vi "test.vi"() -> ()   [LabVIEW 2012]
uses:
  OLD_apparatus_VI/VI/Clearing_mode.ctl
  OLD_apparatus_VI/VI/Readout_mode.ctl
  OLD_apparatus_VI/VI/ADC_gain.ctl
  OLD_apparatus_VI/VI/Image_type.ctl
panel:
  out "Array":T1(array[cluster])
  in  "Image type":T2=7 items=["8 bit signed"=1, "16 bit signed"=2, "32 bit signed"=3, "32 bit floating"=4, "64 bit floating"=5, "8 bit unsigned"=6, "16 bit unsigned"=7, "32 bit unsigned"=8]
  in  "Number of Images":u32=10
  in  "Acquire / Focus Flag":u32=1
  in  "stop":bool=TRUE
  out "Number of Cameras":i32
  out "img":u16[][](graph)
  out "Ydim":u32
  out "Xdim":u32
  out "Camera Handle":u32
  out "error out":errorcluster
  out "Image Handle":u32
  in  "ADC Gain":T3=-1 items=["Use current ADC"=-1, "Use the fastest ADC"=-2, "Use the slowest ADC"=-3]
  in  "FastADC":bool
  in  "ReadoutMode":T4=2.0 caption="Readout Mode" items=["Normal readout"=1.0, "Frame transfer readout"=2.0, "MPP readout"=3.0, "Frame transfer MPP"=4.0, "Alternate timing for normal readout"=5.0, "Alternate timing for frame transfer"=6.0, "Alternate timing for MPP"=7.0, "Alternate timing for frame transfer MPP"=8.0, "Interline"=9.0]
  in  "ClearMode":T5=1.0 caption="Clearing Mode" items=["Clear never"=1.0, "Clear pre-exposure"=2.0, "Clear pre-sequence"=3.0, "Clear post-sequence"=4.0, "Clear pre- and post-sequence"=5.0, "Clear pre-exposure and post-sequence"=6.0]
  in  "EMGain":dbl=3500.0 caption="EM Gain" format="%.2f"
  in  "Exposure (sec)":dbl=0.01 format="%.3f"
  in  "Temperature":dbl=-70.0 format="%.2f"
  in  "error in (no error)":errorcluster
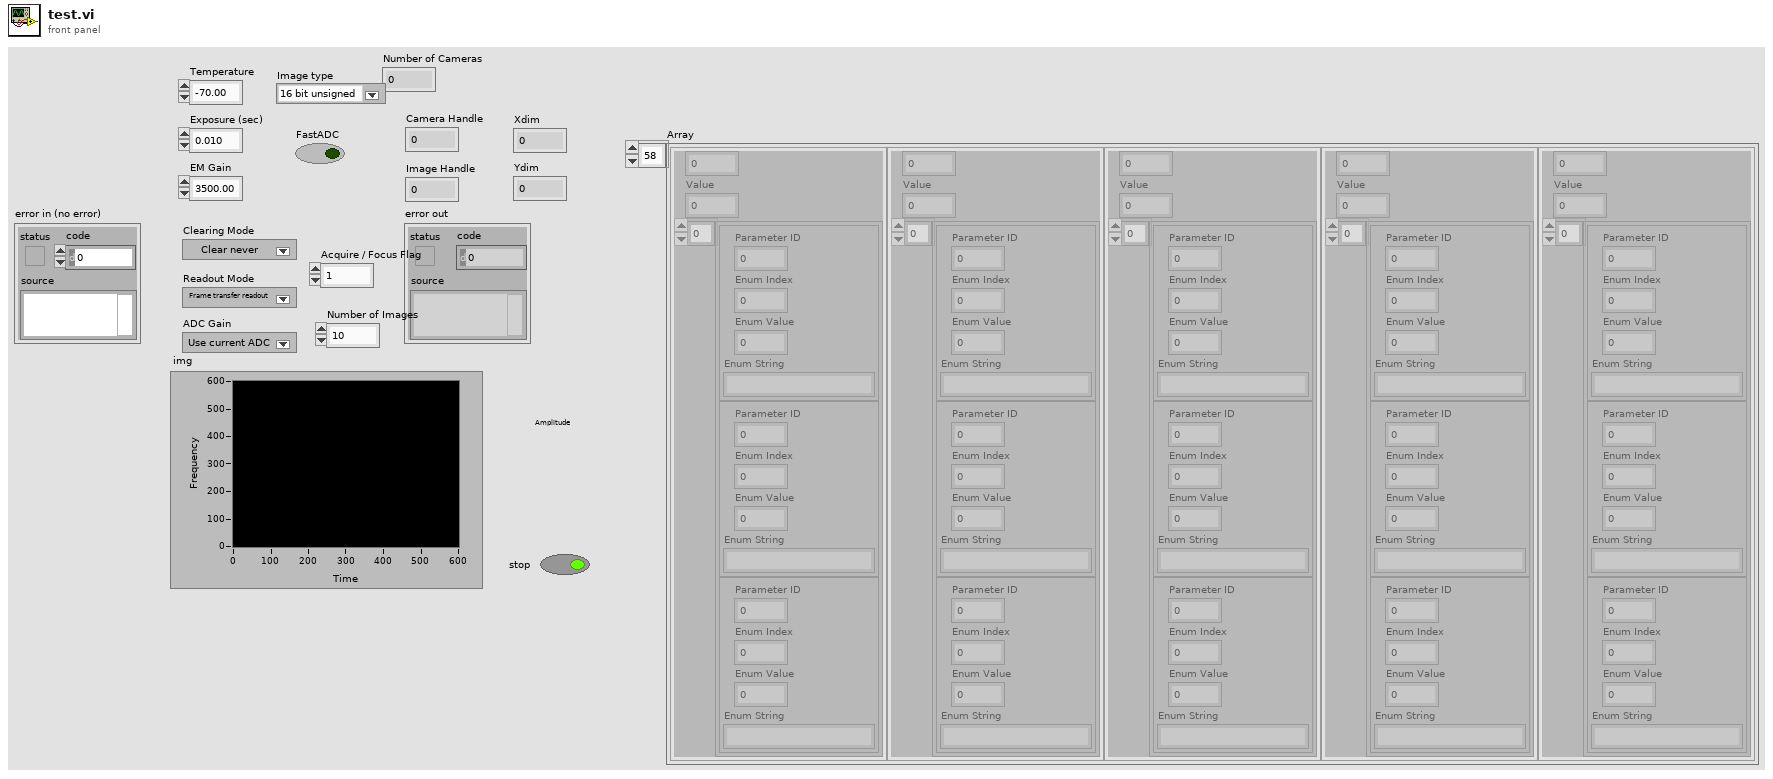
[diagram p1: front panel]
types:
  T1 = cluster{i32, "Value":dbl, cluster{"Parameter ID":u32, "Enum Index":u32, "Enum Value":dbl, "Enum String":string}[]}[]
  T2 = typedef "Image_type.ctl" = u32
  T3 = typedef "ADC_gain.ctl" = i32
  T4 = typedef "Readout_mode.ctl" = dbl
  T5 = typedef "Clearing_mode.ctl" = dbl
  T6 = cluster{"Parameter ID":u32, "Enum Index":u32, "Enum Value":dbl, "Enum String":string}
  T7 = cluster{i32, "Value":dbl, cluster{"Parameter ID":u32, "Enum Index":u32, "Enum Value":dbl, "Enum String":string}[]}
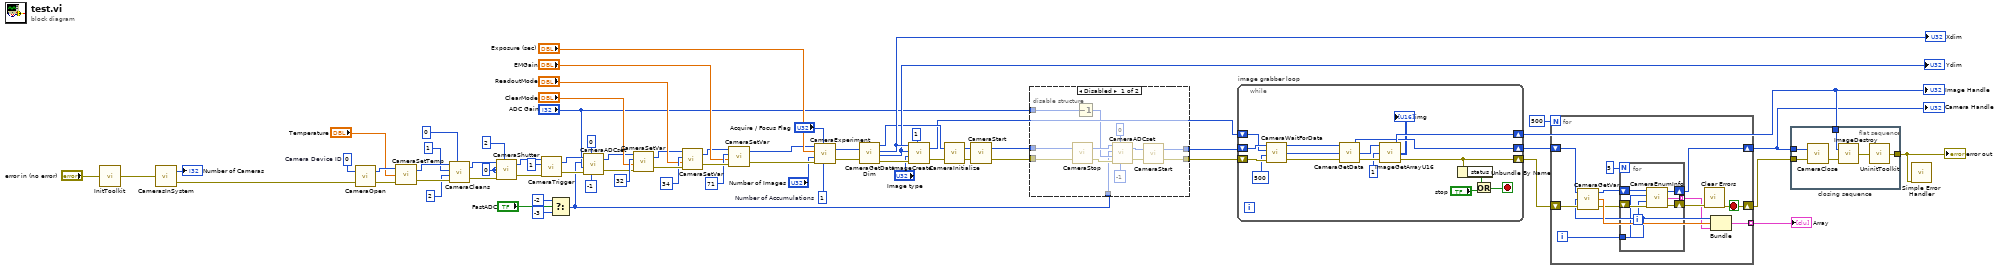
[diagram p0: block diagram]
diagram:
  w14 = u32 1  # Number of Accumulations
  w70 = u32 0  # Camera Device ID
  w60 = u32 0 ("Shutter Comp Time: Pre Open")
  n1 = call <userlib>:"InitToolkit.vi"("error in"="error in (no error)") -> ("error out"=w20:errorcluster)
  n2 = call <userlib>:"CamerasInSystem.vi"("error in"=w20) -> ("Number of Cameras"=→"Number of Cameras":i32, "error out"=w19:errorcluster)
  n3 = call <userlib>:"CameraOpen.vi"("error in"=w19, "Camera Device ID"=w70) -> ("error out"=w68:errorcluster, "Camera Handle"=w69:u32)
  n4 = call <userlib>:"CameraSetTemp.vi"("error in (no error)"=w68, "Temperature"="Temperature", "Camera Handle"=w69) -> ("error out"=w64:errorcluster, "Camera Handle"=w63:u32)
  n5 = call <userlib>:"CameraCleans.vi"("Camera Handle"=w63, "Number of Clears"=u32 1, "Number of Strips Per Clear"=u32 2, "error in"=w64, "Continuous Clears"=u32 0) -> ("Camera Handle"=w65:u32, "error out"=w66:errorcluster)
  n6 = call <userlib>:"CameraShutter.vi"("Camera Handle"=w65, "Shutter Comp Time: Pre Open"=w60, "Shutter Comp Time: Post Open"=w60, "error in"=w66, "Shutter State"=u32 2) -> ("Camera Handle"=w57:u32, "error out"=w58:errorcluster)
  n7 = call <userlib>:"CameraTrigger.vi"("error in"=w58, "Timing Mode"=u32 1, "Camera Handle"=w57) -> ("error out"=w43:errorcluster, "Camera Handle"=w44:u32)  [unwired: 1 in]
  n8 = Select(t=-2 ("Fastest\nADC"), s="FastADC", f=-3 ("Slowest\nADC")) -> (s? t:f=w22:i32)
  n9 = call <userlib>:"CameraADCset.vi"("ADC offset"=-1, "Read Out port"=0, "error in (no error)"=w43, "ADC Gain"="ADC Gain", "ADC Speed"=w22, "Camera Handle"=w44) -> ("error out"=w42:errorcluster, "Camera Handle"=w41:u32)
  n10 = call <userlib>:"CameraSetVar.vi"("error in"=w42, "Value"="ClearMode", "Parameter ID"=u32 32, "Camera Handle"=w41) -> ("error out"=w51:errorcluster, "CameraHandle"=w32:u32)
  n11 = call <userlib>:"CameraSetVar.vi"("error in"=w51, "Value"="ReadoutMode", "Parameter ID"=u32 34, "Camera Handle"=w32) -> ("error out"=w47:errorcluster, "CameraHandle"=w31:u32)
  n12 = call <userlib>:"CameraSetVar.vi"("error in"=w47, "Value"="EMGain", "Parameter ID"=u32 71, "Camera Handle"=w31) -> ("error out"=w38:errorcluster, "CameraHandle"=w37:u32)
  n13 = call <userlib>:"CameraExperiment.vi"("Number of Accumulations"=w14, "Acquire / Focus Flag"="Acquire / Focus Flag", "error in"=w38, "Number of Images"="Number of Images", "Exposure (sec)"="Exposure (sec)", "Camera Handle"=w37) -> ("error out"=w55:errorcluster, "Camera Handle"=w10:u32)
  n14 = call <userlib>:"CameraGetDataDim.vi"("Camera Handle"=w10, "error in"=w55) -> ("Camera Handle"=w9:u32, "Xdim"=w34:u32, "Ydim"=w33:u32, "error out"=w36:errorcluster)
  "Xdim" <- w34
  "Ydim" <- w33
  n15 = call <userlib>:"ImageCreate.vi"("X dimension"=w34, "Y dimension"=w33, "Data Type"="Image type", "error in"=w36, "Number Of Frames"=u32 1) -> ("Image Handle"=w7:u32, "error out"=w12:errorcluster)
  n16 = call <userlib>:"CameraInitialize.vi"("error in"=w12, "Camera Handle"=w9) -> ("error out"=w11:errorcluster, "Camera Handle"=w13:u32)
  n17 = call <userlib>:"CameraStart.vi"("error in"=w11, "Camera Handle"=w13) -> ("error out"=w27:errorcluster, "Camera Handle"=w26:u32)
  n18 = disable-structure shown="Disabled" {
    disable-tunnel: w27 -> [w80 w85]
    disable-tunnel: w26 -> [w79 w86]
    disable-tunnel: [w78 w85] -> w25
    disable-tunnel: [w77 w86] -> w24
    disable-tunnel: "ADC Gain" -> [w74 _]
    disable-tunnel: w22 -> [w72 _]
    frame Disabled {
      n19 = call <userlib>:"CameraStop.vi"("error in"=w80, "Camera Handle"=w79) -> ("error out"=w81:errorcluster, "Camera Handle"=w82:u32)
      n20 = Decrement(x=w74) -> (x-1=w73:T3)
      n21 = call <userlib>:"CameraADCset.vi"("ADC offset"=-1, "Read Out port"=0, "error in (no error)"=w81, "ADC Gain"=w73, "ADC Speed"=w72, "Camera Handle"=w82) -> ("error out"=w76:errorcluster, "Camera Handle"=w75:u32)
      n22 = call <userlib>:"CameraStart.vi"("error in"=w76, "Camera Handle"=w75) -> ("error out"=w78:errorcluster, "Camera Handle"=w77:u32)
    }
    frame Enabled {
    }
  }
  n23 = while "image grabber loop" {
    shift-right: [w102] -> w21
    shift-left: w7 -> [w93]
    shift-right: [w101] -> w6
    shift-left: w24 -> [w97]
    shift-right: [w103] -> w4
    shift-left: w25 -> [w96]
    stop <- w99 stop-if-true
    n24 = call <userlib>:"CameraWaitForData.vi"("error in"=w96, "Time Out ms"=u32 500, "Image Handle"=w93, "Camera Handle"=w97) -> ("error out"=w95:errorcluster, "Image Handle"=w92:u32, "Camera Handle"=w94:u32)
    n25 = call <userlib>:"CameraGetData.vi"("error in"=w95, "Data Handle"=w92, "Camera Handle"=w94) -> ("error out"=w90:errorcluster, "Data Handle"=w89:u32, "Camera Handle"=w101:u32)
    n26 = call <userlib>:"ImageGetArrayU16.vi"("error in"=w90, "Z position"=u32 1 ("Z Position"), "Image Handle"=w89) -> ("error out"=w103:errorcluster, "Array uint 16"=→"img":u16[][], "Image Handle"=w102:u32)
    n27 = Unbundle By Name(w103) -> ("status"=w100:bool)
    n28 = Or(x=w100, y="stop") -> (x .or. y?=w99:bool)
  }
  "Image Handle" <- w21
  n29 = for {
    N: 500 -> [_]
    shift-right: [w111] -> w3
    shift-left: w4 -> [w114]
    shift-right: [w109] -> w5
    shift-left: w6 -> [w115]
    tunnel: [w112] -> w1 mode=indexing
    i -> [w106]
    stop <- w111 stop-if-true
    n30 = call <userlib>:"CameraGetVar.vi"("error in"=w114, "Parameter ID"=w106, "Camera Handle"=w115) -> ("error out"=w108:errorcluster, "Value"=w113:dbl, "Camera Handle"=w110:u32)
    n31 = for {
      N: 5 -> [_]
      tunnel: w106 -> [w118]
      tunnel: [w117] -> w105 mode=indexing
      shift-right: [w121] -> w109
      shift-left: w110 -> [w122]
      shift-right: [w119] -> w107
      shift-left: w108 -> [w120]
      i -> [w116]
      n32 = call <userlib>:"CameraEnumInfo.vi"("error in"=w120, "Enum Index"=w116, "Parameter ID"=w118, "Camera Handle"=w122) -> ("error out"=w119:errorcluster, "Enum Information"=w117:T6, "Camera Handle"=w121:u32)
    }
    n33 = call <vilib>:"Clear Errors.vi"("error in (no error)"=w107) -> ("error out"=w111:errorcluster)  [unwired: 6 in]
    n34 = Bundle(w106, "Value"=w113, w105) -> (w112:T7)  [unwired: 1 in]
  }
  "Camera Handle" <- w5
  "Array" <- w1
  n35 = flat-sequence "closing sequence" {
    tunnel: w5 -> [w126]
    tunnel: w21 -> [w125]
    tunnel: w3 -> [w124]
    tunnel: [w123] -> w17
    frame #0 {
      n36 = call <userlib>:"CameraClose.vi"("error in"=w124, "Camera Handle"=w126) -> ("error out"=w127:errorcluster)
      n37 = call <userlib>:"ImageDestroy.vi"("error in"=w127, "Data handle"=w125) -> ("error out"=w128:errorcluster)
      n38 = call <userlib>:"UninitToolkit.vi"("error in"=w128) -> ("error out"=w123:errorcluster)
    }
  }
  n39 = call <vilib>:"Simple Error Handler.vi"("error in (no error)"=w17) -> ()  [unwired: 4 in, 5 out]
  "error out" <- w17
